vi "InitializeCamera.vi"() -> (0 "error out":errorcluster, 1 "EM Gain Range":i32[](array[numeric]), 2 "EM Speeds":string[](array[string]), 3 "exposure time":sgl=0.1, 4 "ypixels":i32, 5 "xpixels":i32, 7 "EM Gain":u32)   [LabVIEW 2015]
uses:
  <userlib>/atmcd64d.llb/AcquisitionMode_mode typedef.ctl
  <userlib>/atmcd64d.llb/ReadMode_mode typedef.ctl
  <userlib>/atmcd64d.llb/TriggerMode_mode typedef.ctl
  <userlib>/atmcd64d.llb/Shutter_type typedef.ctl
  <userlib>/atmcd64d.llb/Shutter_mode typedef.ctl
  <userlib>/atmcd64d.llb/HSSpeed_type typedef.ctl
  LiveImage_Global.vi
panel:
  out "error out 2":errorcluster
  out "#VS Speeds":i32
  out "minTemp":i32
  out "maxTemp":i32
  out "temperature":sgl
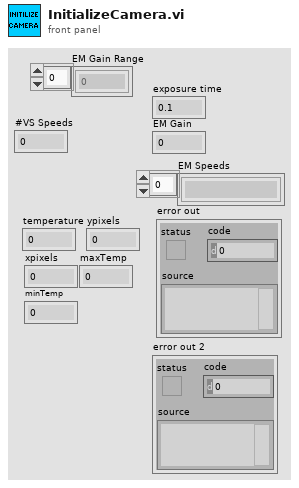
[diagram p1: front panel]
types:
  T1 = typedef "HSSpeed_type typedef.ctl" = enum16{"EM Amp", "Conventional Amp"}
  T2 = typedef "Shutter_mode typedef.ctl" = enum16{"Auto", "Open", "Close", "N/A (3)", "Open FVB Series", "Open Any Series"}
  T3 = typedef "Shutter_type typedef.ctl" = enum16{"TTL Low", "TTL High"}
  T4 = typedef "TriggerMode_mode typedef.ctl" = enum16{"Internal", "External", "N/A (2)", "N/A (3)", "N/A (4)", "N/A (5)", "External Start", "External Exposure (Bulb)", "N/A (8)", "External FVB EM", "Software", "N/A (11)", "External Charge Shifting"}
  T5 = typedef "ReadMode_mode typedef.ctl" = enum16{"Full Vertical Binning", "Multi-Track", "Random-Track", "Single-Track", "Image"}
  T6 = typedef "AcquisitionMode_mode typedef.ctl" = enum16{"Reserved (0)", "Single Scan", "Accumulate", "Kinetics", "Fast Kinetics", "Run Till Abort", "Reserved (6)", "Reserved (7)", "Reserved (8)", "Time Delayed Integration"}
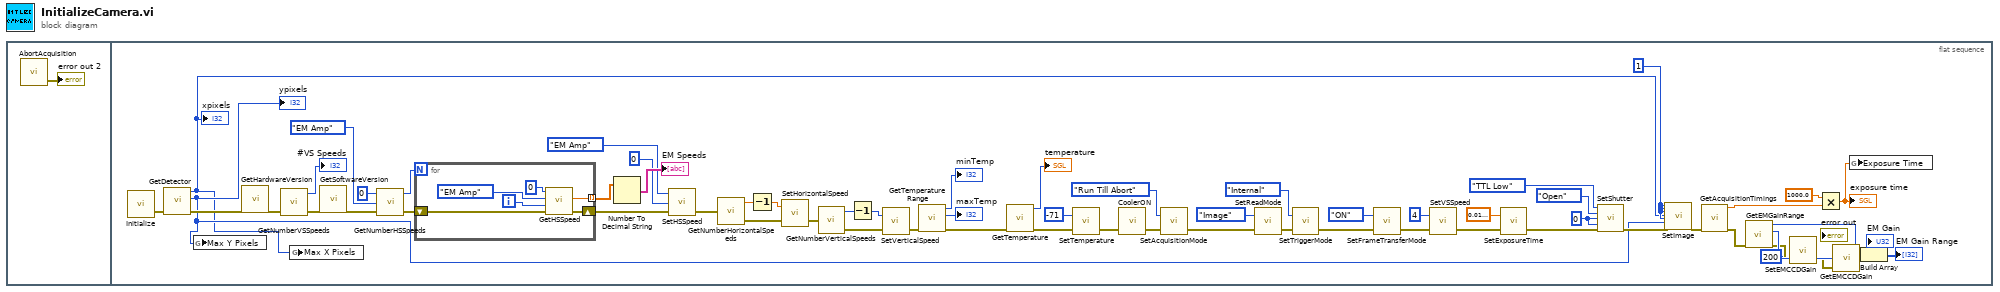
[diagram p0: block diagram]
diagram:
  n1 = flat-sequence {
    frame #0 {
      n2 = call <userlib>:"AbortAcquisition.vi"() -> ("error out"=→"error out 2":errorcluster)  [unwired: 2 in, 1 out]
    }
    frame #1 {
      w35 = 0 ("closingtime")
      w39 = 1 ("hbin")
      n3 = call <userlib>:"Initialize.vi"() -> ("error out"=w63:errorcluster)  [unwired: 2 in, 1 out]
      n4 = call <userlib>:"GetDetector.vi"("error in (no error)"=w63) -> ("error out"=w62:errorcluster, "ypixels"=w11:i32, "xpixels"=w10:i32)  [unwired: 3 in, 1 out]
      "xpixels" <- w10
      "ypixels" <- w11
      n5 = global write "LiveImage_Global.vi" "Max Y Pixels"(w11) -> ()
      n6 = call <userlib>:"GetHardwareVersion.vi"("error in (no error)"=w62) -> ("error out"=w61:errorcluster)  [unwired: 19 in, 7 out]
      n7 = call <userlib>:"GetNumberVSSpeeds.vi"("error in (no error)"=w61) -> ("error out"=w60:errorcluster, "number"=→"#VS Speeds":i32)  [unwired: 2 in, 1 out]
      n8 = global write "LiveImage_Global.vi" "Max X Pixels"(w10) -> ()
      n9 = call <userlib>:"GetSoftwareVersion.vi"("error in (no error)"=w60) -> ("error out"=w54:errorcluster)  [unwired: 19 in, 7 out]
      n10 = call <userlib>:"GetNumberHSSpeeds.vi"("error in (no error)"=w54, "type"=HSSpeed_type_typedef."EM Amp", "channel"=0) -> ("error out"=w53:errorcluster, "number"=w52:i32)  [unwired: 1 out]
      n11 = for {
        N: w52 -> [_]
        tunnel: [w69] -> w45 mode=indexing
        shift-right: [w67] -> w25
        shift-left: w53 -> [w70]
        i -> [w68]
        n12 = call <userlib>:"GetHSSpeed.vi"("error in (no error)"=w70, "index"=w68, "type"=HSSpeed_type_typedef."EM Amp", "channel"=0) -> ("error out"=w67:errorcluster, "speed"=w69:sgl)  [unwired: 1 in, 1 out]
      }
      n13 = Number To Decimal String(number=w45) -> (decimal integer string=→"EM Speeds":string[])  [unwired: 1 in]
      n14 = call <userlib>:"SetHSSpeed.vi"("error in (no error)"=w25, "index"=0, "type"=HSSpeed_type_typedef."EM Amp") -> ("error out"=w20:errorcluster)  [unwired: 1 in, 1 out]
      n15 = call <userlib>:"GetNumberHorizontalSpeeds.vi"("error in (no error)"=w20) -> ("number"=w19:dbl, "error out"=w18:errorcluster)  [unwired: 1 out]
      n16 = Decrement(x=w19) -> (x-1=w17:dbl)
      n17 = call <userlib>:"SetHorizontalSpeed.vi"("error in (no error)"=w18, "index"=w17) -> ("error out"=w13:errorcluster)  [unwired: 1 out]
      n18 = call <userlib>:"GetNumberVerticalSpeeds.vi"("error in (no error)"=w13) -> ("number"=w15:i32, "error out"=w16:errorcluster)  [unwired: 1 out]
      n19 = Decrement(x=w15) -> (x-1=w14:i32)
      n20 = call <userlib>:"SetVerticalSpeed.vi"("error in (no error)"=w16, "index"=w14) -> ("error out"=w12:errorcluster)  [unwired: 1 out]
      n21 = call <userlib>:"GetTemperatureRange.vi"("error in (no error)"=w12) -> ("error out"=w57:errorcluster, "maxTemp"=→"maxTemp":i32, "minTemp"=→"minTemp":i32)  [unwired: 3 in, 1 out]
      n22 = call <userlib>:"GetTemperature.vi"("error in (no error)"=w57) -> ("error out"=w51:errorcluster, "temperature"=→"temperature":i32)  [unwired: 3 in, 2 out]
      n23 = call <userlib>:"SetTemperature.vi"("error in (no error)"=w51, "temperature"=-71) -> ("error out"=w50:errorcluster)  [unwired: 1 out]
      n24 = call <userlib>:"CoolerON.vi"("error in (no error)"=w50) -> ("error out"=w48:errorcluster)  [unwired: 1 in, 1 out]
      n25 = call <userlib>:"SetAcquisitionMode.vi"("error in (no error)"=w48, "mode"=AcquisitionMode_mode_typedef."Run Till Abort") -> ("error out"=w42:errorcluster)  [unwired: 1 out]
      n26 = call <userlib>:"SetReadMode.vi"("error in (no error)"=w42, "mode"=ReadMode_mode_typedef."Image") -> ("error out"=w30:errorcluster)  [unwired: 1 out]
      n27 = call <userlib>:"SetTriggerMode.vi"("error in (no error)"=w30, "mode"=TriggerMode_mode_typedef."Internal") -> ("error out"=w33:errorcluster)  [unwired: 1 out]
      n28 = call <userlib>:"SetFrameTransferMode.vi"("error in (no error)"=w33, "mode"=enum16{"OFF", "ON"}."ON") -> ("error out"=w31:errorcluster)  [unwired: 1 out]
      n29 = call <userlib>:"SetVSSpeed.vi"("error in (no error)"=w31, "index"=4) -> ("error out"=w40:errorcluster)  [unwired: 1 out]
      n30 = call <userlib>:"SetExposureTime.vi"("error in (no error)"=w40, "time"=sgl 0.02) -> ("error out"=w38:errorcluster)  [unwired: 1 out]
      n31 = call <userlib>:"SetShutter.vi"("type"=Shutter_type_typedef."TTL Low", "mode"=Shutter_mode_typedef."Open", "closingtime"=w35, "openingtime"=w35, "error in (no error)"=w38) -> ("error out"=w29:errorcluster)  [unwired: 9 in, 1 out]
      n32 = call <userlib>:"SetImage.vi"("hbin"=w39, "vbin"=w39, "hstart"=w39, "hend"=w10, "vstart"=w39, "vend"=w11, "error in (no error)"=w29) -> ("error out"=w22:errorcluster)  [unwired: 19 in, 1 out]
      n33 = call <userlib>:"GetAcquisitionTimings.vi"("error in (no error)"=w22) -> ("exposure"=w21:sgl, "error out"=w9:errorcluster)  [unwired: 10 in, 3 out]
      n34 = call <userlib>:"GetEMGainRange.vi"("error in (no error)"=w9) -> ("error out"=w5:errorcluster, "high"=w8:i32, "low"=w7:i32)  [unwired: 3 in, 1 out]
      n35 = call <userlib>:"SetEMCCDGain.vi"("error in (no error)"=w5, "gain"=200) -> ("error out"=w3:errorcluster)  [unwired: 1 out]
      n36 = Multiply(x=sgl 1000.0, y=w21) -> (x*y=w26:sgl)
      "exposure time" <- w26
      n37 = call <userlib>:"GetEMCCDGain.vi"("error in (no error)"=w3) -> ("gain"=→"EM Gain":u32)  [unwired: 2 in, 2 out]
      n38 = global write "LiveImage_Global.vi" "Exposure Time"(w26) -> ()
      n39 = Build Array(w7, w8) -> (→"EM Gain Range":i32[])
    }
  }
